vi "Read Stimulus Values Scaled.vi"(8 "Error In":errorcluster, 11 "VISA resource name":refnum<visa-resource-name>) -> (0 "Error Out":errorcluster, 1 "Frequency span":T1, 2 "Stimulus List (raw)":dbl[](array[numeric]), 3 "VISA resource name out":refnum<visa-resource-name>)   [LabVIEW 2016]
doc: "This VI for the HP8753B Network Analyzers reads the stimulus values. Except when performing log sweeps and freq list sweeps, this VI uses the start and stop values and the number of points to calcuate the stimulus values."
uses:
  <instrlib>/Agilent 87XX Series/Agilent 87XX Series.lvlib
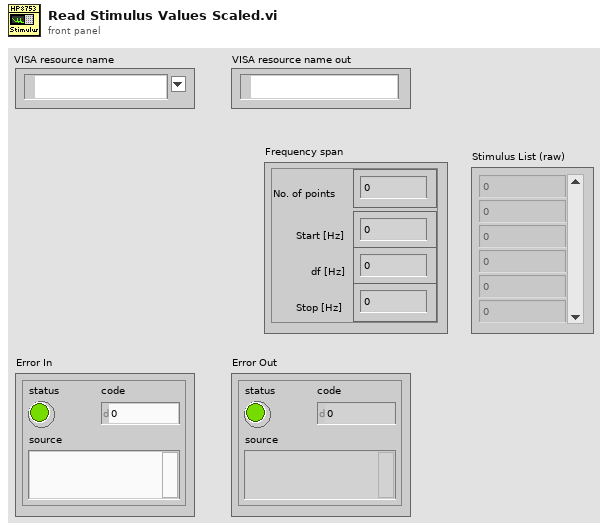
[diagram p1: front panel]
types:
  T1 = cluster{"Start [Hz]":dbl, "No. of points":i32, "df [Hz]":dbl, "Stop [Hz]":dbl}
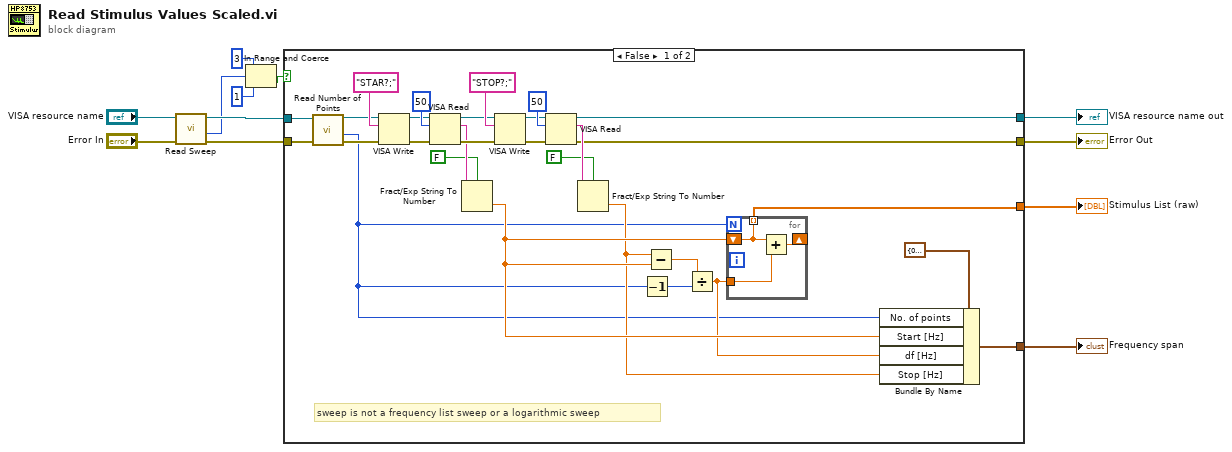
[diagram p0: block diagram]
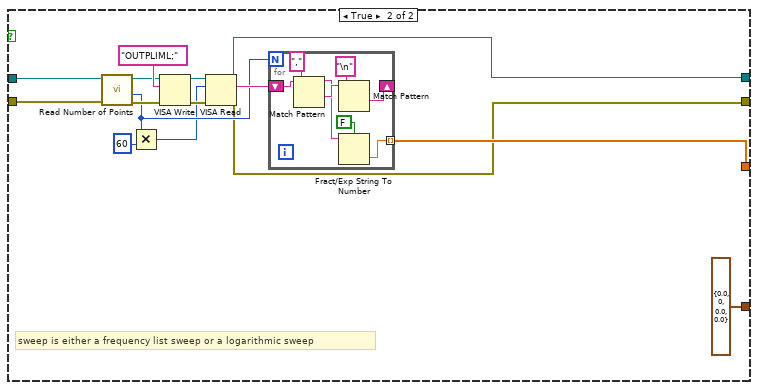
[diagram p2: hidden frame]
diagram:
  n1 = call <instrlib>:"Read Sweep.vi"("error in (no error)"="Error In", "VISA resource name"="VISA resource name") -> ("error out"=w11:errorcluster, "sweep type"=w7:i32, "VISA resource name out"=w12:refnum<visa-resource-name>)  [unwired: 7 in]
  n2 = In Range and Coerce(upper limit=3, x=w7, lower limit=1) -> (In Range?=w10:bool)  [unwired: 1 out]
  n3 = case shown="False" w10 {
    tunnel: w12 -> [w28 w51]
    tunnel: [w31 w55] -> w1
    tunnel: w11 -> [w27 w50]
    tunnel: [w30 w49] -> w2
    tunnel: [w29 w48] -> w4
    tunnel: [w13 T1 {"Start [Hz]"=0.0, "No. of points"=0, "df [Hz]"=0.0, "Stop [Hz]"=0.0} ("Frequency span 2")] -> w6
    frame False {
      # "sweep is not a frequency list sweep or a logarithmic sweep"
      n4 = call <instrlib>:"Read Number of Points.vi"("error in (no error)"=w27, "VISA resource name"=w28) -> ("error out"=w25:errorcluster, "num points"=w14:i32, "VISA resource name out"=w26:refnum<visa-resource-name>)  [unwired: 7 in]
      n5 = VISA Write(VISA resource name=w26, write buffer="STAR?;", error in (no error)=w25) -> (VISA resource name out=w21:refnum<visa-resource-name>, error out=w41:errorcluster)  [unwired: 1 out]
      n6 = VISA Read(VISA resource name=w21, byte count=50, error in (no error)=w41) -> (VISA resource name out=w37:refnum<visa-resource-name>, read buffer=w35:string, error out=w36:errorcluster)  [unwired: 1 out]
      n7 = Fract/Exp String To Number(use system decimal point (T)=FALSE, string=w35) -> (number=w17:dbl)  [unwired: 2 in, 1 out]
      n8 = VISA Write(VISA resource name=w37, write buffer="STOP?;", error in (no error)=w36) -> (VISA resource name out=w22:refnum<visa-resource-name>, error out=w38:errorcluster)  [unwired: 1 out]
      n9 = VISA Read(VISA resource name=w22, byte count=50, error in (no error)=w38) -> (VISA resource name out=w30:refnum<visa-resource-name>, read buffer=w34:string, error out=w29:errorcluster)  [unwired: 1 out]
      n10 = Fract/Exp String To Number(use system decimal point (T)=FALSE, string=w34) -> (number=w15:dbl)  [unwired: 2 in, 1 out]
      n11 = Decrement(x=w14) -> (x-1=w32:i32)
      n12 = Subtract(x=w15, y=w17) -> (x-y=w33:dbl)
      n13 = Divide(x=w33, y=w32) -> (x/y=w16:dbl)
      n14 = for {
        N: w14 -> [_]
        shift-right: [w42] -> _
        shift-left: w17 -> [w44]
        tunnel: w16 -> [w43]
        tunnel: [w44] -> w31 mode=indexing
        n15 = Add(x=w44, y=w43) -> (x+y=w42:dbl)
      }
      n16 = Bundle By Name(cluster=T1 {"Start [Hz]"=0.0, "No. of points"=0, "df [Hz]"=0.0, "Stop [Hz]"=0.0} ("Frequency span 2"), "No. of points"=w14, "Start [Hz]"=w17, "df [Hz]"=w16, "Stop [Hz]"=w15) -> (w13:T1)
    }
    frame True {
      # "sweep is either a frequency list sweep or a logarithmic sweep"
      n17 = call <instrlib>:"Read Number of Points.vi"("error in (no error)"=w50, "VISA resource name"=w51) -> ("error out"=w53:errorcluster, "num points"=w52:i32, "VISA resource name out"=w54:refnum<visa-resource-name>)  [unwired: 7 in]
      n18 = Multiply(x=w52, y=60) -> (x*y=w46:i32)
      n19 = VISA Write(VISA resource name=w54, write buffer="OUTPLIML;", error in (no error)=w53) -> (VISA resource name out=w47:refnum<visa-resource-name>, error out=w59:errorcluster)  [unwired: 1 out]
      n20 = VISA Read(VISA resource name=w47, byte count=w46, error in (no error)=w59) -> (VISA resource name out=w49:refnum<visa-resource-name>, read buffer=w58:string, error out=w48:errorcluster)  [unwired: 1 out]
      n21 = for {
        N: w52 -> [_]
        shift-right: [w63] -> _
        shift-left: w58 -> [w67]
        tunnel: [w61] -> w55 mode=indexing
        n22 = Match Pattern(string=w67, regular expression=",") -> (before substring=w62:string, after substring=w65:string)  [unwired: 1 in, 2 out]
        n23 = Match Pattern(string=w65, regular expression="\n") -> (after substring=w63:string)  [unwired: 1 in, 3 out]
        n24 = Fract/Exp String To Number(use system decimal point (T)=FALSE, string=w62) -> (number=w61:dbl)  [unwired: 2 in, 1 out]
      }
    }
  }
  "Frequency span" <- w6
  "Error Out" <- w4
  "VISA resource name out" <- w2
  "Stimulus List (raw)" <- w1
